vi "CallFacialClassFunction_LVPic.vi"(8 "error in (no error)":errorcluster, 9 "Function or Method Name":string="findFaces", 10 "image":picture, 11 "reference in":refnum<class "ImageFacialDetection.lvclass">) -> (0 "error out":errorcluster, 2 "image with faces":picture, 3 "reference out":refnum<class "ImageFacialDetection.lvclass">)   [LabVIEW 2017, in "ImageFacialDetection.lvclass"]
doc: "uses the image classification in python with openCV to detect faces in an image using Haar Cascades"
uses:
  ImageFacialDetection.lvclass
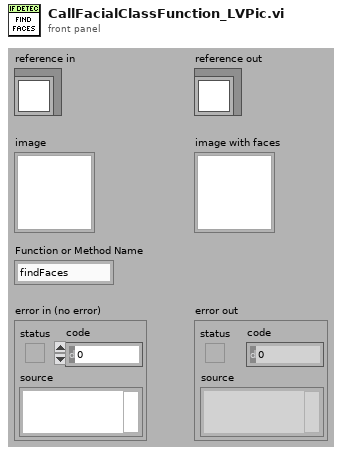
[diagram p1: front panel]
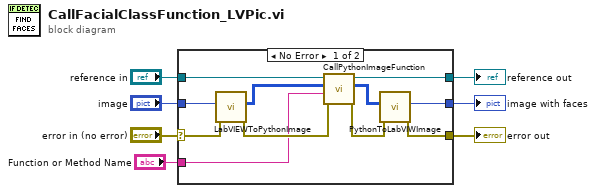
[diagram p0: block diagram]
diagram:
  n1 = case shown="No Error" "error in (no error)" {
    selector: "error in (no error)" -> [w12 w20]
    tunnel: [w9 w20] -> w6
    tunnel: [w17 w19] -> w4
    tunnel: "reference in" -> [w18 w19]
    tunnel: "image" -> [w16 _]
    tunnel: [w13 _] -> w2
    tunnel: "Function or Method Name" -> [w8 _]
    frame No Error {
      n2 = call "LabVIEWToPythonImage.vi"("error in (no error)"=w12, "image"=w16) -> ("error out"=w11:errorcluster, "Python Image Data"=w14:u8[][][])  [unwired: 8 in]
      n3 = call "CallPythonImageFunction.vi"("error in (no error)"=w11, "Function or Method Name"=w8, "Python Image Data in"=w14, "reference in"=w18) -> ("error out"=w10:errorcluster, "Python Image Data out"=w15:u8[][][], "reference out"=w17:refnum<class "ImageFacialDetection.lvclass">)  [unwired: 5 in]
      n4 = call "PythonToLabVIWImage.vi"("error in (no error)"=w10, "Python Image"=w15) -> ("error out"=w9:errorcluster, "LabVIEW Picture"=w13:picture)  [unwired: 8 in]
    }
    frame Error {
    }
  }
  "error out" <- w6
  "reference out" <- w4
  "image with faces" <- w2
